vi "光源散斑模块.vi"(2 "图像信息簇":T1, 3 "采样次数":i32, 4 "模块调用信息簇":T3) -> (0 "光源散斑簇":T2)   [LabVIEW 2018]
uses:
  <vilib>/imath/engines/lvmath2/RunTimeEngine/BuiltInFunctions/rand/NIMS_rand(1,I32).vi
  <vilib>/imath/engines/lvmath2/RunTimeEngine/ErrorHandling/NIMS_Error From Error Code.vi
  <vilib>/imath/engines/lvmath2/RunTimeEngine/BuiltInFunctions/sum/NIMS_sum(GV).vi
  <instcachedir>/0/NIMS_sum(GV)_67F5EC36BC034E54A6BEC5B0673C00E5.lvgen/NIMS_sum(GV)_67F5EC36BC034E54A6BEC5B0673C00E5_000.vi
  <vilib>/imath/engines/lvmath2/RunTimeEngine/NodeEndStatement/NIMS_NodeEndStatement_Output.vi
  <instcachedir>/0/NIMS_NodeEndStatement_Output_53EC0D466D134D7ABD903AC30B43404B.lvgen/NIMS_NodeEndStatement_Output_53EC0D466D134D7ABD903AC30B43404B_005.vi
  <vilib>/imath/engines/lvmath2/RunTimeEngine/ErrorHandling/NIMS_Finalize Error.vi
panel:
  out "输出数组":dbl[](array[numeric])
  out "转置的矩阵":dbl[][](array[numeric])
  out "数组 3":dbl[][](array[numeric])
  out "数组":sgl[][](array[numeric])
  out "appended path":path=path "F:/Hadamard_simulation/dmd"
  out "piexls of pattern":i32=4096
  out "采样进度":u8(slide)=100 scale=0.0..100.0
  out "error out":errorcluster
  out "初始化的数组 2":dbl[](array[numeric])
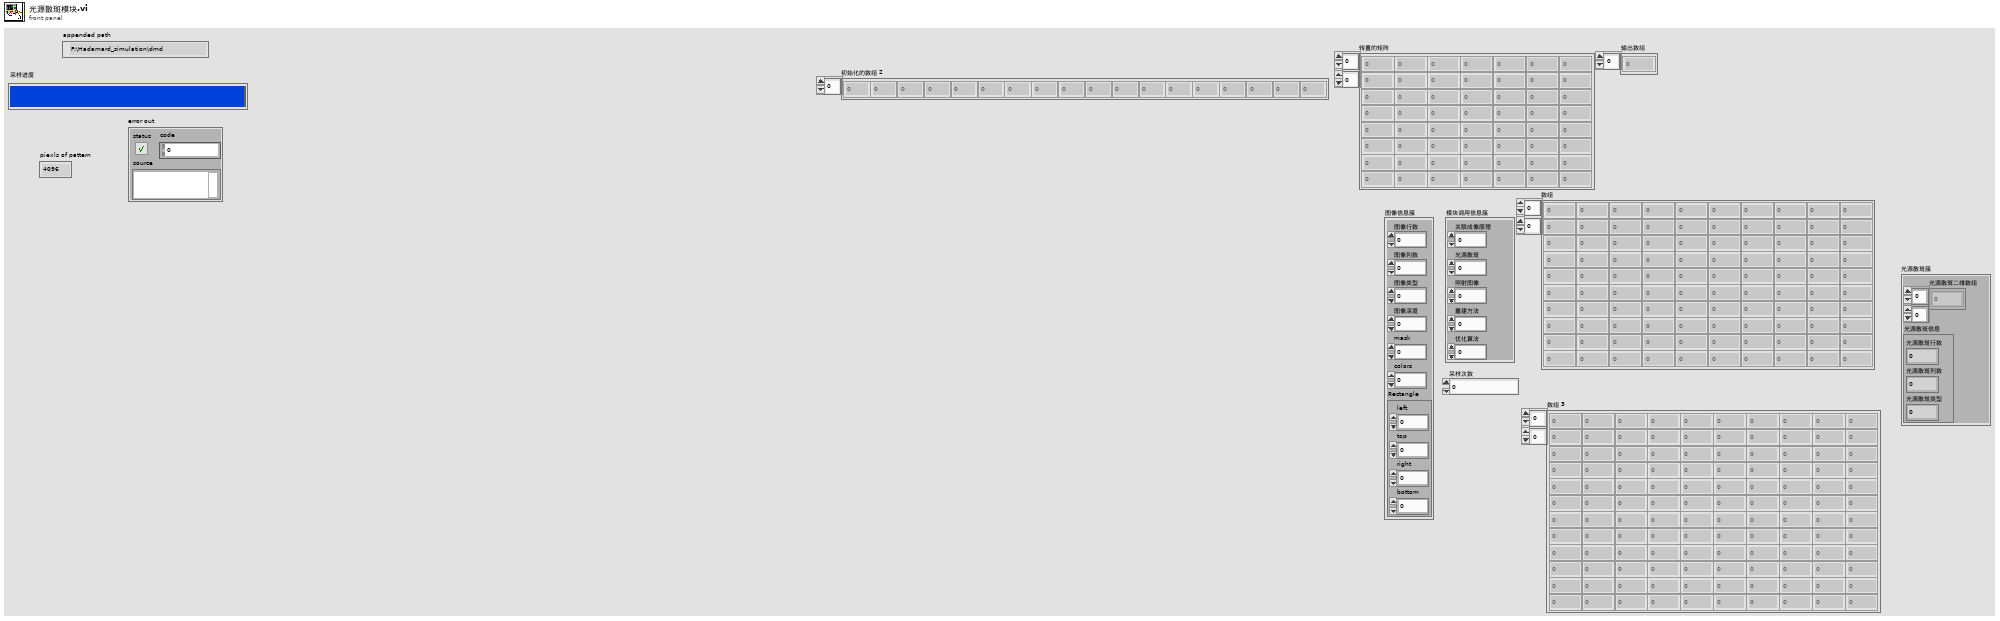
[diagram p1: front panel]
types:
  T1 = cluster{"图像行数":dbl, "图像列数":dbl, "图像类型":dbl, "图像深度":i32, "mask":i32, "colors":i32, "Rectangle":cluster{"left":i16, "top":i16, "right":i16, "bottom":i16}}
  T2 = cluster{"光源散斑二维数组":dbl[][], "光源散斑信息":cluster{"光源散斑行数":dbl, "光源散斑列数":dbl, "光源散斑类型":dbl}}
  T3 = cluster{"关联成像原理":i32, "光源散斑":i32, "照射图像":i32, "重建方法":i32, "优化算法":i32}
  T4 = enum16{"open", "replace", "create", "open or create", "replace or create", "replace or create with confirmation"}
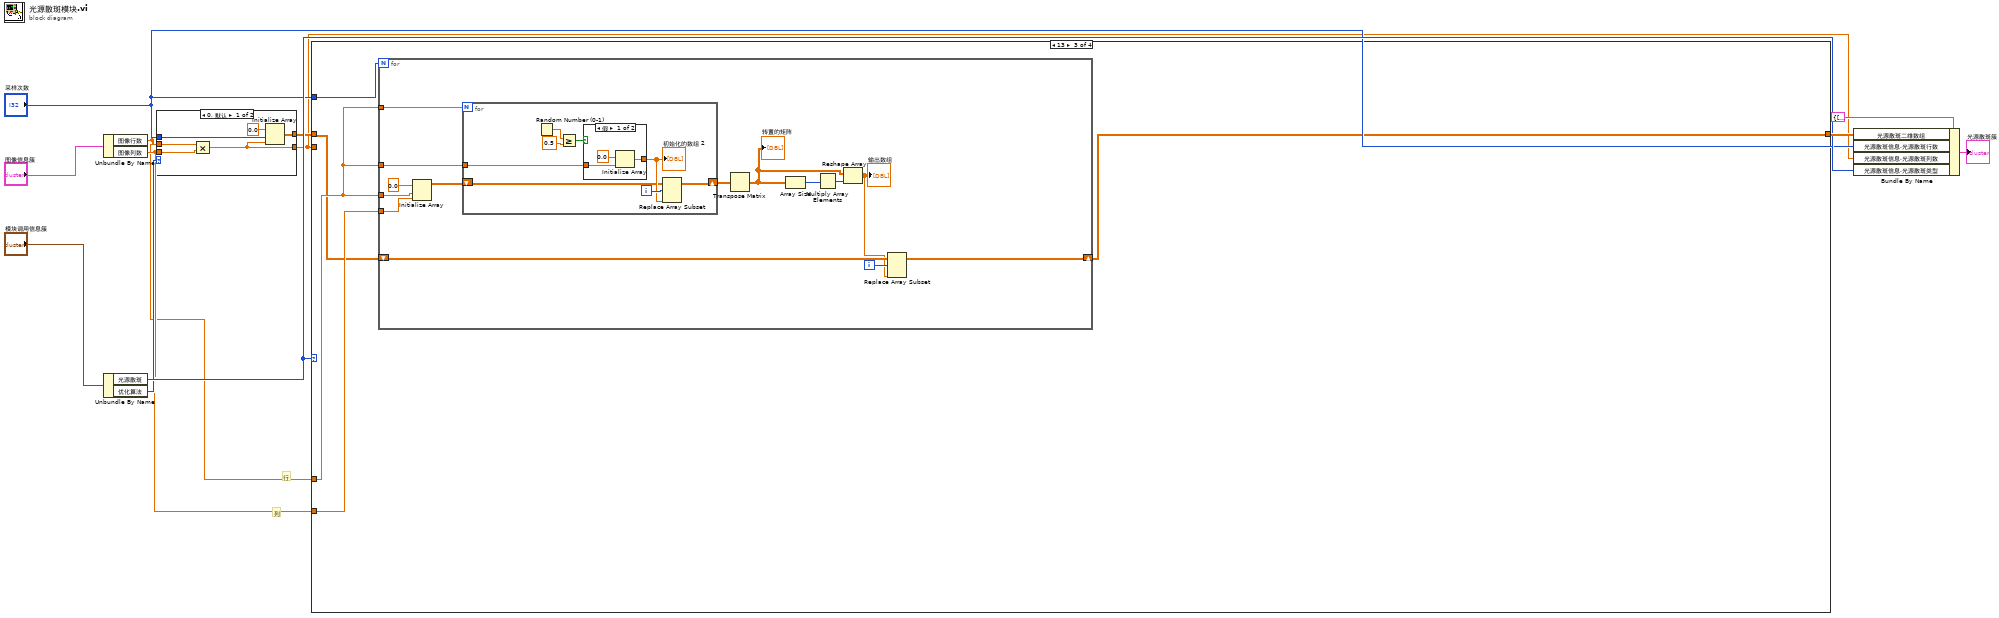
[diagram p0: block diagram]
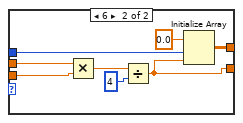
[diagram p2: hidden frame]
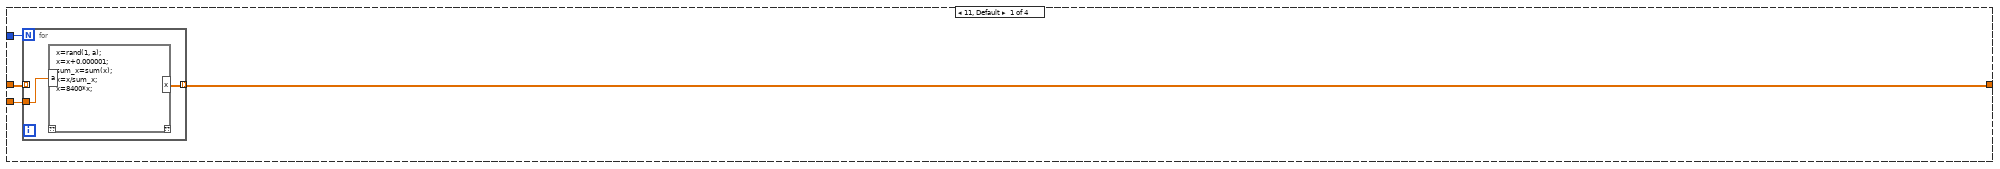
[diagram p3: hidden frame]
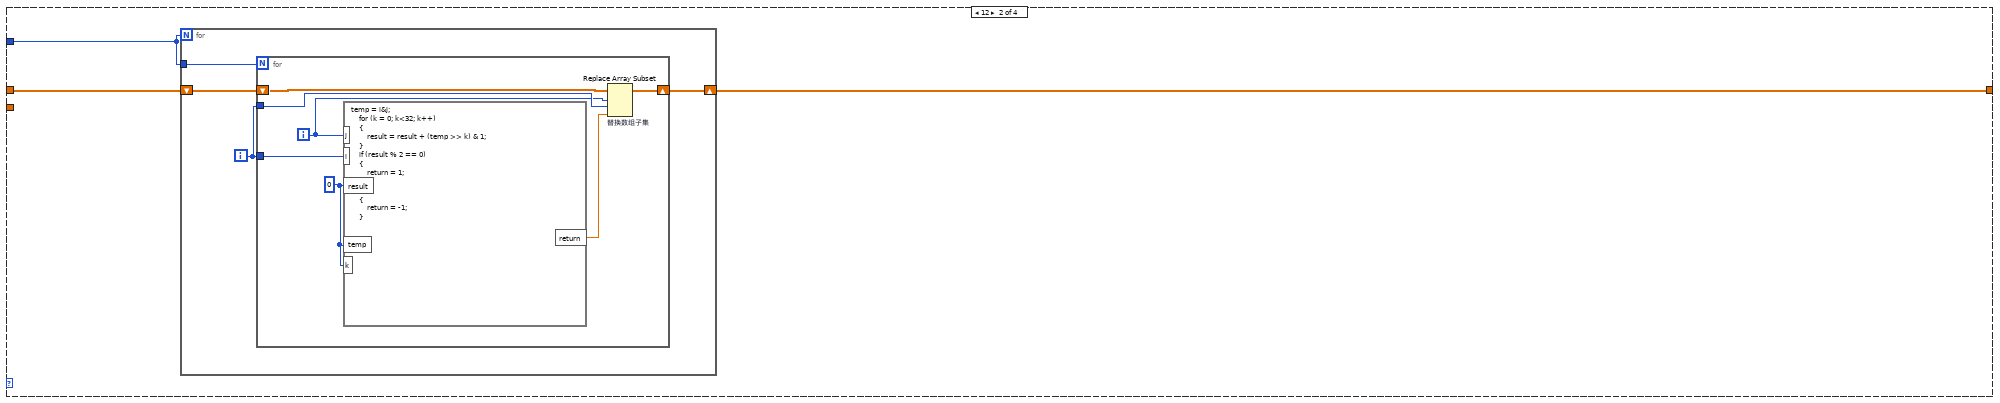
[diagram p4: hidden frame]
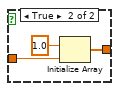
[diagram p5: hidden frame]
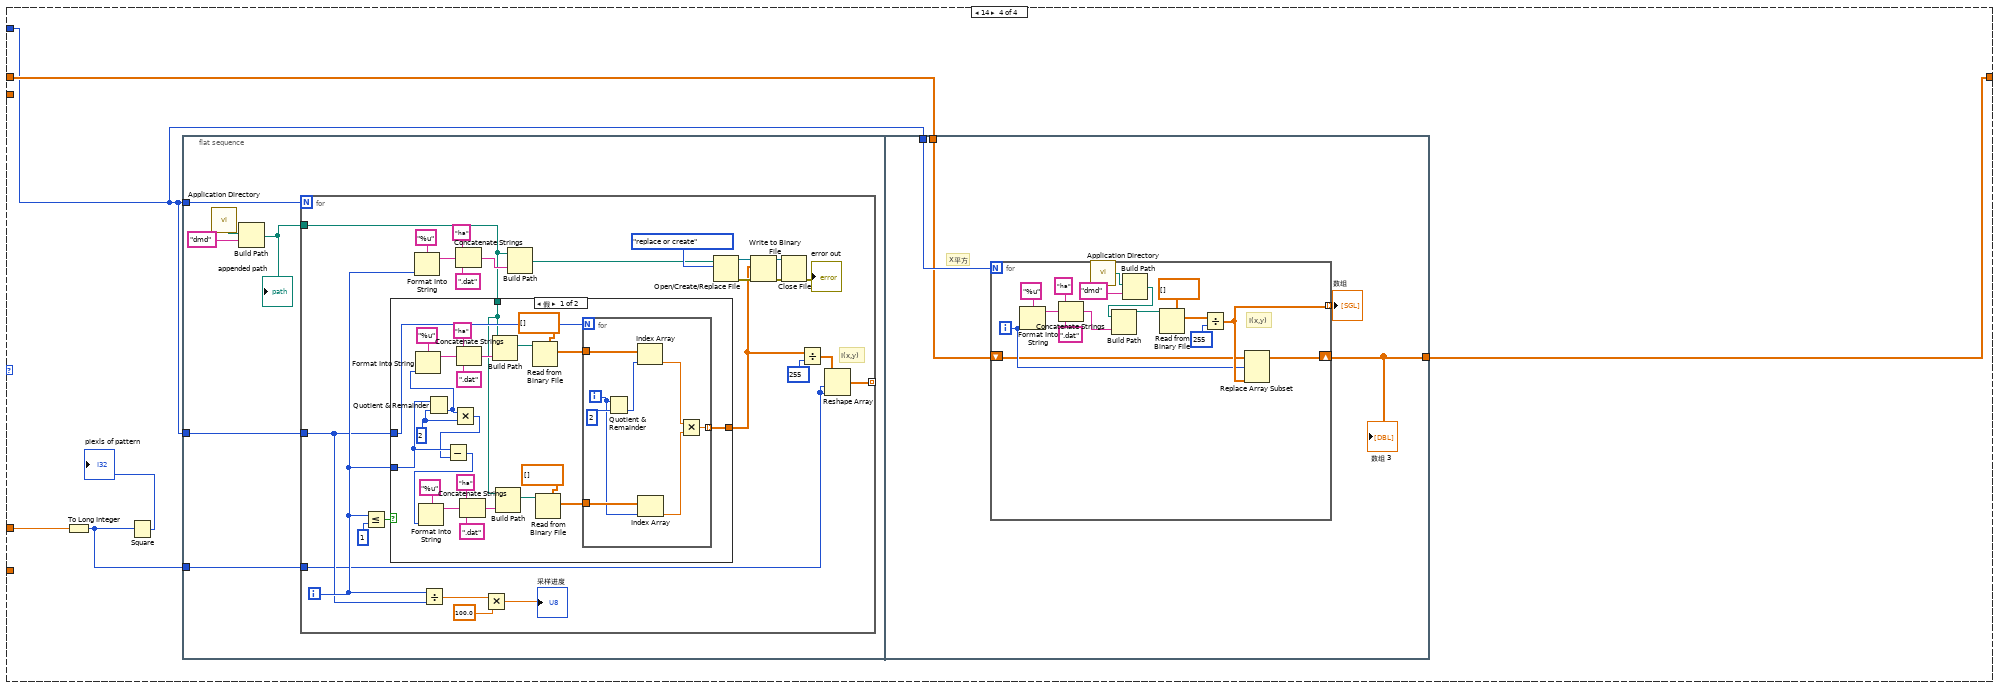
[diagram p6: hidden frame]
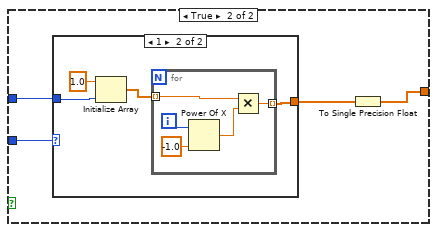
[diagram p7: hidden frame]
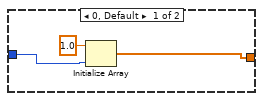
[diagram p8: hidden frame]
diagram:
  # "列"
  # "行"
  n1 = Unbundle By Name("图像信息簇") -> ("图像行数"=w1:dbl, "图像列数"=w2:dbl)
  n2 = Unbundle By Name("模块调用信息簇") -> ("光源散斑"=w8:i32, "优化算法"=w6:i32)
  n3 = case shown="0, 默认" w6 {
    tunnel: "采样次数" -> [w18 w24]
    tunnel: [w17 w25] -> w4
    tunnel: w2 -> [w15 w22]
    tunnel: w1 -> [w14 w23]
    tunnel: [w13 w19] -> w3
    frame 0, Default {
      n4 = Multiply(x=w14, y=w15) -> (x*y=w13:dbl)
      n5 = Initialize Array(0.0, w18, w13) -> (w17:dbl[][])
    }
    frame 6 {
      n6 = Multiply(x=w23, y=w22) -> (x*y=w21:dbl)
      n7 = Divide(x=w21, y=4) -> (x/y=w19:dbl)
      n8 = Initialize Array(0.0, w24, w19) -> (w25:dbl[][])
    }
  }
  n9 = case shown="13" w8 {
    tunnel: "采样次数" -> [w30 w91 w106 w137]
    tunnel: w4 -> [w28 w90 w105 w139]
    tunnel: [w29 w92 w104 w138] -> w11
    tunnel: w3 -> [w27 _ _ _]
    tunnel: w1 -> [_ _ w107 w142]
    tunnel: w2 -> [_ _ w108 _]
    frame 11, Default {
      n10 = for {
        N: w30 -> [_]
        tunnel: [w31] -> w29 mode=indexing
        tunnel: w28 -> [_] mode=indexing
        tunnel: w27 -> [w32]
        n11 = mathscript code="x=rand(1, a);\nx=x+0.000001;\nsum_x=sum(x);\nx=x/sum_x;\nx=8400*x;"("a"=w32) -> ("x"=w31:dbl[])  [unwired: 1 in, 1 out]
      }
    }
    frame 12 {
      n12 = for {
        N: w91 -> [_]
        shift-right: [w94] -> w92
        shift-left: w90 -> [w96]
        tunnel: w91 -> [w93]
        i -> [w95]
        n13 = for {
          N: w93 -> [_]
          shift-right: [w99] -> w94
          shift-left: w96 -> [w102]
          tunnel: w95 -> [w101]
          tunnel: w95 -> [w100]
          i -> [w98]
          w103 = 0
          n14 = formula code="temp = i&j;\n    for (k = 0; k<32; k++)\n    {\n        result = result + (temp >> k) & 1;\n    }\n    if (result % 2 == 0)\n    {\n        return = 1;\n    }\n    else\n    {\n        return = -1;\n    }"("result"=w103, "temp"=w103, "k"=w103, "i"=w101, "j"=w98) -> ("return"=w97:dbl)
          n15 = Replace Array Subset "替换数组子集"(array=w102, new element=w97, index (row)=w98, index (col)=w100) -> (w99:dbl[][])
        }
      }
    }
    frame 13 {
      n16 = for {
        N: w106 -> [_]
        tunnel: w107 -> [w116]
        tunnel: w108 -> [w115]
        tunnel: w107 -> [w114]
        tunnel: w107 -> [w113]
        shift-right: [w111] -> w104
        shift-left: w105 -> [w112]
        i -> [w110]
        n17 = Initialize Array(0.0 ("元素"), w116, w115) -> (w118:dbl[][])
        n18 = for {
          N: w114 -> [_]
          tunnel: w113 -> [w125]
          shift-right: [w123] -> w119
          shift-left: w118 -> [w124]
          i -> [w130]
          n19 = Random Number (0-1)() -> (number: 0 to 1=w128:dbl)
          n20 = Greater Or Equal?(x=w128, y=0.5) -> (x >= y?=w129:bool)
          n21 = case shown="假" w129 {
            tunnel: [w132 w135] -> w126
            tunnel: w125 -> [w131 w134]
            frame False {
              n22 = Initialize Array(0.0 ("元素"), w131) -> (w132:dbl[])
            }
            frame True {
              n23 = Initialize Array(1.0 ("元素"), w134) -> (w135:dbl[])
            }
          }
          "初始化的数组 2" <- w126
          n24 = Replace Array Subset(array=w124, new element=w126, index (row)=w130) -> (w123:dbl[][])  [unwired: 1 in]
        }
        n25 = Transpose Matrix(1:w119) -> (0:w122:dbl[][])
        "转置的矩阵" <- w122
        n26 = Array Size(array=w122) -> (size(s)=w120:i32[])
        n27 = Multiply Array Elements(1:w120) -> (0:w121:i32)
        n28 = Reshape Array(w122, w121) -> (w109:dbl[])
        "输出数组" <- w109
        n29 = Replace Array Subset(array=w112, new element=w109, index (row)=w110) -> (w111:dbl[][])  [unwired: 1 in]
      }
    }
    frame 14 {
      n30 = To Long Integer(number=w142) -> (32bit integer=w141:i32)
      n31 = Square(x=w141) -> (x^2=→"piexls of pattern":i32)
      n32 = flat-sequence {
        tunnel: w137 -> [w145]
        tunnel: w137 -> [w144]
        tunnel: w141 -> [w143]
        tunnel: w137 -> [w225]
        tunnel: w139 -> [w223]
        tunnel: [w222] -> w138
        frame #0 {
          n33 = call <vilib>:"Application Directory.vi"() -> ("Application Directory"=w147:path)
          n34 = Build Path(base path=w147, name or relative path="dmd") -> (appended path=w148:path)
          "appended path" <- w148
          n35 = for {
            N: w145 -> [_]
            tunnel: w144 -> [w156]
            tunnel: w148 -> [w154]
            tunnel: [w150] -> _ mode=indexing
            tunnel: w143 -> [w149]
            i -> [w164]
            # "I(x,y)"
            n36 = Less Or Equal?(x=w164, y=1 ("元素")) -> (x <= y?=w165:bool)
            n37 = case shown="假" w165 {
              tunnel: w164 -> [w189 w209]
              tunnel: w156 -> [w197 w208]
              tunnel: [w174 w206] -> w151
              tunnel: w154 -> [w177 _]
              frame False {
                w188 = 2 ("y")
                n38 = Quotient & Remainder(x=w189, y=w188) -> (floor(x/y)=w186:i32)  [unwired: 1 out]
                n39 = Format Into String(format string="%u" ("格式字符串"), w186) -> (resulting string=w194:string)  [unwired: 2 in, 1 out]
                n40 = Multiply(x=w186, y=w188) -> (x*y=w187:i32)
                n41 = Subtract(x=w189, y=w187) -> (x-y=w178:i32)
                n42 = Format Into String(format string="%u" ("格式字符串"), w178) -> (resulting string=w183:string)  [unwired: 2 in, 1 out]
                n43 = Concatenate Strings("ha" ("字符串"), w194, ".dat" ("字符串")) -> (w191:string)
                n44 = Concatenate Strings("ha" ("字符串"), w183, ".dat" ("字符串")) -> (w180:string)
                n45 = Build Path(base path=w177, name or relative path=w191) -> (appended path=w196:path)
                n46 = Build Path(base path=w177, name or relative path=w180) -> (appended path=w185:path)
                n47 = Read from Binary File(5:sgl[] [], 11:w196) -> (2:w176:sgl[])  [unwired: 1 in, 6 out]
                n48 = Read from Binary File(5:sgl[] [], 11:w185) -> (2:w175:sgl[])  [unwired: 1 in, 6 out]
                n49 = for {
                  N: w197 -> [_]
                  tunnel: w176 -> [w204]
                  tunnel: w175 -> [w202]
                  tunnel: [w198] -> w174 mode=indexing
                  i -> [w201]
                  n50 = Quotient & Remainder(x=w201, y=2) -> (floor(x/y)=w203:i32)  [unwired: 1 out]
                  n51 = Index Array(array=w204, index=w203) -> (element=w200:sgl)
                  n52 = Index Array(array=w202, index=w201) -> (element=w199:sgl)
                  n53 = Multiply(x=w200, y=w199) -> (x*y=w198:sgl)
                }
              }
              frame True {
                n54 = case shown="1" w209 {
                  tunnel: w208 -> [w211 w215]
                  tunnel: [w210 w213] -> w207
                  frame 0, Default {
                    n55 = Initialize Array(1.0 ("元素"), w211) -> (w210:dbl[])
                  }
                  frame 1 {
                    n56 = Initialize Array(1.0 ("元素"), w215) -> (w214:dbl[])
                    n57 = for {
                      tunnel: w214 -> [w221] mode=indexing
                      tunnel: [w217] -> w213 mode=indexing
                      i -> [w219]
                      n58 = Power Of X(1:-1.0 ("元素"), 2:w219) -> (0:w218:dbl)
                      n59 = Multiply(x=w221, y=w218) -> (x*y=w217:dbl)
                    }
                  }
                }
                n60 = To Single Precision Float(number=w207) -> (single precision float=w206:sgl[])
              }
            }
            n61 = Format Into String(format string="%u" ("格式字符串"), w164) -> (resulting string=w167:string)  [unwired: 2 in, 1 out]
            n62 = Divide(x=w164, y=w156) -> (x/y=w173:dbl)
            n63 = Concatenate Strings("ha" ("字符串"), w167, ".dat" ("字符串")) -> (w170:string)
            n64 = Multiply(x=w173, y=100.0) -> (x*y=→"采样进度":dbl)
            n65 = Build Path(base path=w154, name or relative path=w170) -> (appended path=w157:path)
            n66 = Open/Create/Replace File(file path (use dialog)=w157, operation (0:open)=T4."replace or create") -> (refnum out=w160:refnum<file>, error out=w159:errorcluster)  [unwired: 4 in, 1 out]
            n67 = Write to Binary File(file (use dialog)=w160, data=w151, error in=w159) -> (refnum out=w161:refnum<file>, error out=w162:errorcluster)  [unwired: 3 in, 1 out]
            n68 = Close File(refnum=w161, error in=w162) -> (error out=→"error out":errorcluster)  [unwired: 1 out]
            n69 = Divide(x=w151, y=255) -> (x/y=w152:sgl[])
            n70 = Reshape Array(w152, w149, w149) -> (w150:sgl[][])
          }
        }
        frame #1 {
          # "X平方"
          n71 = for {
            N: w225 -> [_]
            tunnel: [w229] -> w224 mode=indexing
            shift-right: [w226] -> w222
            shift-left: w223 -> [w227]
            i -> [w228]
            # "I(x,y)"
            n72 = Format Into String(format string="%u" ("格式字符串"), w228) -> (resulting string=w238:string)  [unwired: 2 in, 1 out]
            n73 = Concatenate Strings("ha" ("字符串"), w238, ".dat" ("字符串")) -> (w241:string)
            n74 = call <vilib>:"Application Directory.vi"() -> ("Application Directory"=w231:path)
            n75 = Build Path(base path=w231, name or relative path="dmd") -> (appended path=w230:path)
            n76 = Build Path(base path=w230, name or relative path=w241) -> (appended path=w235:path)
            n77 = Read from Binary File(5:sgl[] [], 11:w235) -> (2:w234:sgl[])  [unwired: 1 in, 6 out]
            n78 = Divide(x=w234, y=255) -> (x/y=w229:sgl[])
            n79 = Replace Array Subset(array=w227, new element=w229, index (row)=w228) -> (w226:dbl[][])  [unwired: 1 in]
          }
          "数组" <- w224
          "数组 3" <- w222
        }
      }
    }
  }
  n80 = Bundle By Name(cluster=T2 {"光源散斑二维数组"=[], "光源散斑信息"={"光源散斑行数"=0.0, "光源散斑列数"=0.0, "光源散斑类型"=0.0}}, "光源散斑二维数组"=w11, "光源散斑信息.光源散斑行数"="采样次数", "光源散斑信息.光源散斑列数"=w3, "光源散斑信息.光源散斑类型"=w8) -> (→"光源散斑簇":T2)
